vi "cupStateGlobal.vi"() -> ()   [LabVIEW 2011]
panel:
  out "CupState":bool
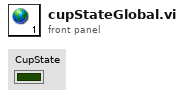
[diagram p1: front panel]
diagram:
